vi "Data_Save_summary.vi"(8 "Data in":T1, 11 "AllControls In":T2) -> (2 "数组":string[](array[string]), 3 "dup path":path)   [LabVIEW 2017]
uses:
  Ctrls/AllControls.ctl
  Ctrls/CSV_Data.ctl
  Ctrls/PathChoose.ctl
  <vilib>/Utility/file.llb/Write Delimited Spreadsheet (string).vi
  <vilib>/Utility/file.llb/Read Delimited Spreadsheet (string).vi
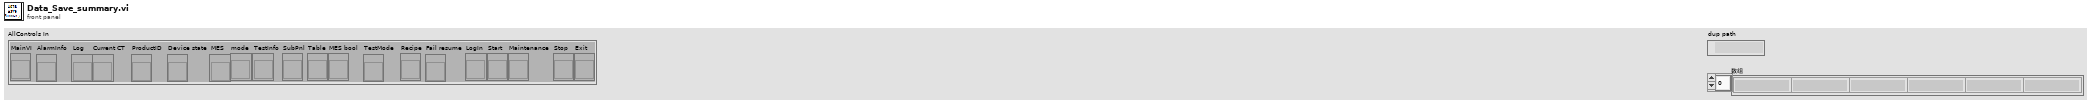
[diagram p1: front panel]
types:
  T1 = typedef "CSV_Data.ctl" = cluster{"SN":string, "Table":string[][], "Count":cluster{"Total":i32, "OK":i32, "NG":i32, "Yield":dbl}, "Start Time":timestamp, "daemon reference":refnum<k5>, "CT":dbl, "OK/NG":bool, "Station ID":string, "MES DDM SN":string, "MES PCBA SN":string, "Retest":string, "Attachment RFID detection":cluster{"UID":string, "tag content":string}, "SKU":string, "Plate_Diameter":string, "Alarm":string}
  T2 = typedef "AllControls.ctl" = cluster{"MainVI":refnum<vi>, "AlarmInfo":refnum<vi>, "Log":refnum<vi>, "Current CT":refnum<vi>, "ProductID":refnum<vi>, "Device state":refnum<vi>, "MES":refnum<vi>, "mode":refnum<vi>, "TestInfo":refnum<vi>, "SubPnl":refnum<vi>, "Table":refnum<vi>, "MES bool":refnum<vi>, "TestMode":refnum<vi>, "Recipe":refnum<vi>, "Fail resume":refnum<vi>, "LogIn":refnum<vi>, "Start":refnum<vi>, "Maintenance":refnum<vi>, "Stop":refnum<vi>, "Exit":refnum<vi>}
  T3 = typedef "PathChoose.ctl" = enum16{"OperatorLog", "AutoRunLog", "AlmLog", "TestData", "AllTestData", "backup_nvm", "backup_before_flashing"}
  T4 = enum16{"open", "replace", "create", "open or create", "replace or create", "replace or create with confirmation"}
  T5 = typedef "TesterInfo.ctl" = cluster{"Station Name":string, "Station Code":string, "ES NO.":string, "Tester ID":string, "PassMark Revision":string, "Rig ID":string, "Deamon_vision":string, "Project Name":string, "FFTesterPath":path, "Enable_User":bool, "Mode":enum16{"682"}, "MES":bool}
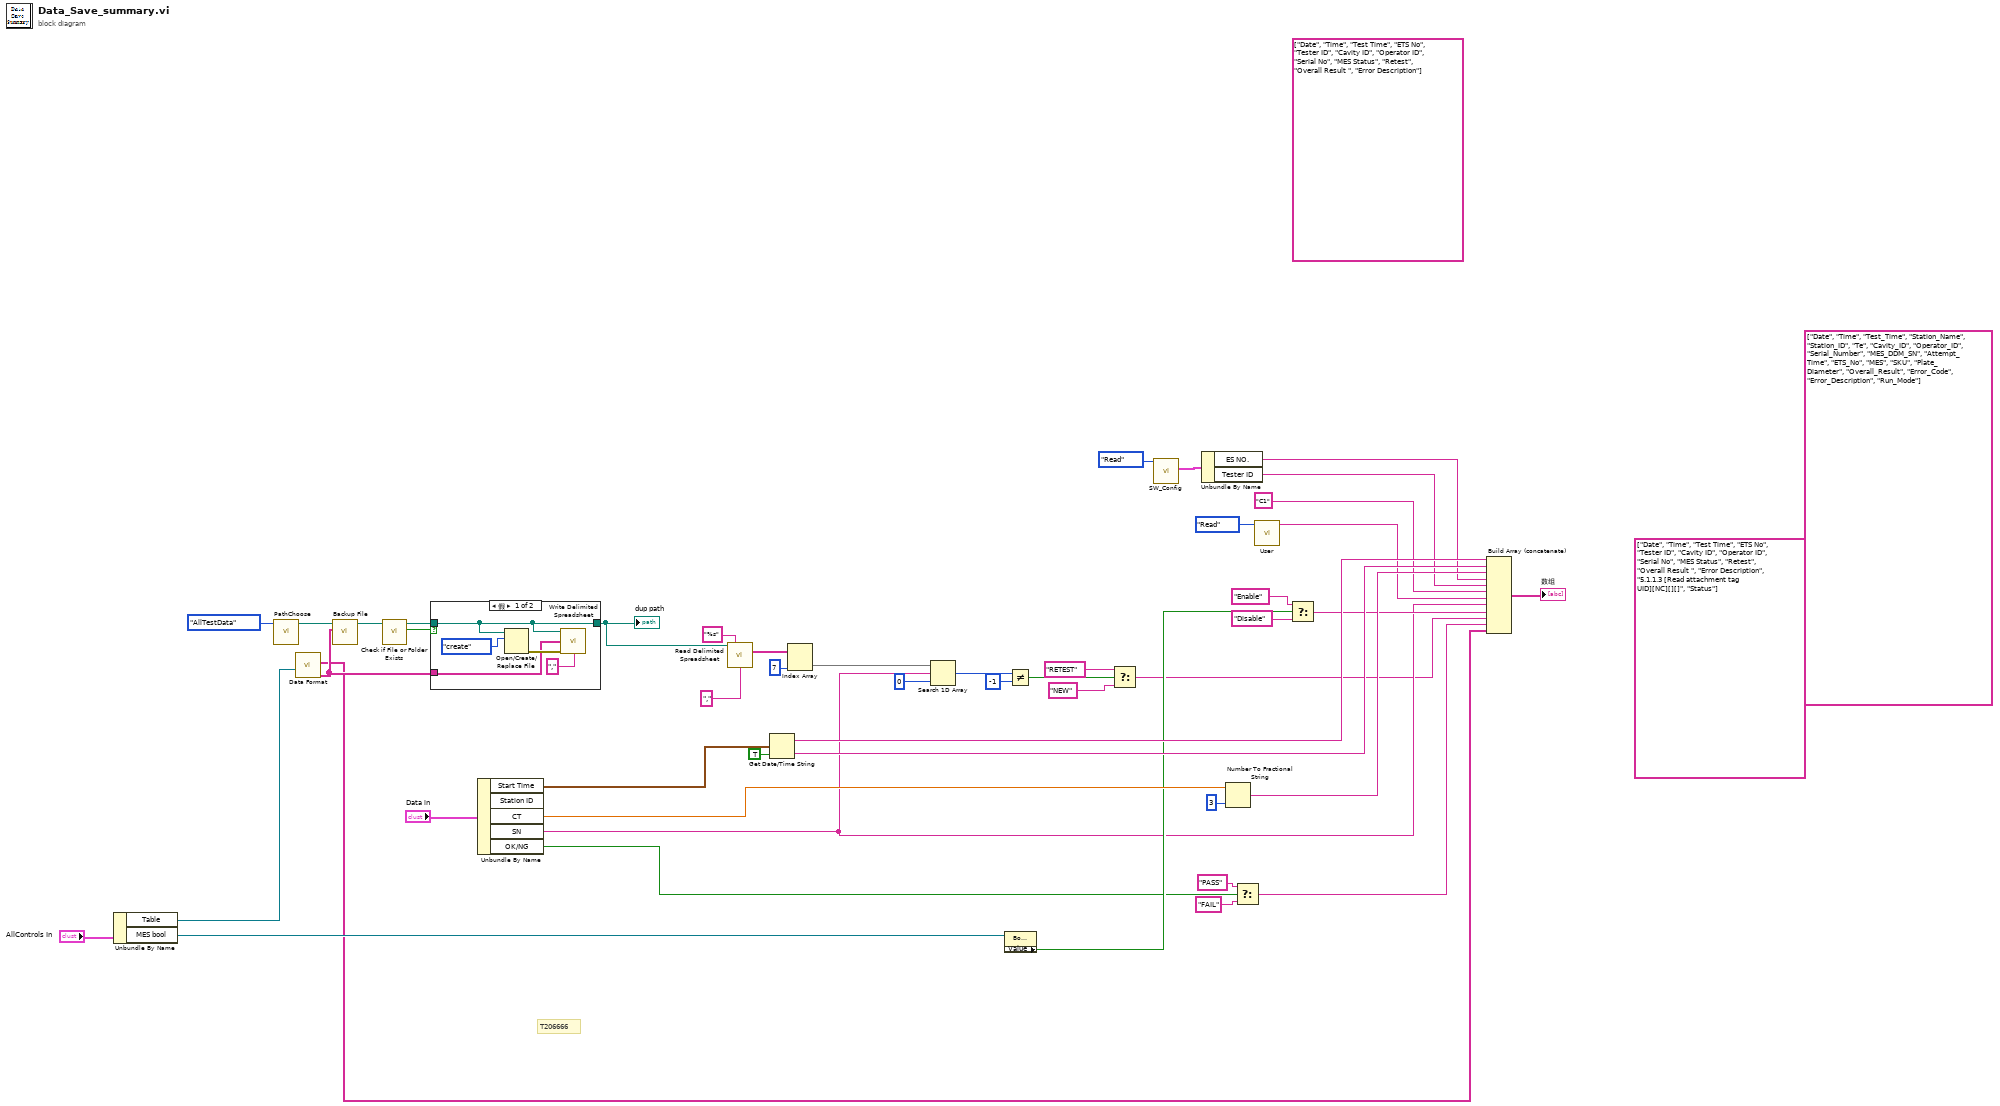
[diagram p0: block diagram]
diagram:
  (unwired) string[] ["Date", "Time", "Test Time", "ETS No", "Tester ID", "Cavity ID", "Operator ID", "Serial No", "MES Status", "Retest", "Overall Result ", "Error Description", "5.1.1.3 [Read attachment tag UID][NC][][]", "Status"] ("title")
  (unwired) string[] ["Date", "Time", "Test Time", "ETS No", "Tester ID", "Cavity ID", "Operator ID", "Serial No", "MES Status", "Retest", "Overall Result ", "Error Description"] ("title")
  (unwired) string[] ["Date", "Time", "Test_Time", "Station_Name", "Station_ID", "Te", "Cavity_ID", "Operator_ID", "Serial_Number", "MES_DDM_SN", "Attempt_Time", "ETS_No", "MES", "SKU", "Plate_Diameter", "Overall_Result", "Error_Code", "Error_Description", "Run_Mode"]
  # "T206666"
  n1 = Unbundle By Name("AllControls In") -> ("Table"=w2:refnum<vi>, "MES bool"=w41:refnum<vi>)
  n2 = call "PathChoose.vi"(11:PathChoose."AllTestData") -> ("Path_Out"=w39:path)  [unwired: 10 in]
  n3 = call "Data Format.vi"("Table"=w2) -> ("title"=w36:string[], "Data"=w1:string[])  [unwired: 9 in]
  n4 = call "Backup File.vi"("列首字符串"=w36, "path"=w39) -> ("path 2"=w38:path)  [unwired: 9 in]
  n5 = call <vilib>:"Check if File or Folder Exists.vi"("path"=w38) -> ("file or folder exists?"=w47:bool, "dup path"=w46:path)  [unwired: 8 in, 1 out]
  n6 = case shown="假" w47 {
    tunnel: w46 -> [w51 w54]
    tunnel: [w51 w54] -> w13
    tunnel: w36 -> [w49 _]
    frame False {
      n7 = Open/Create/Replace File(file path (use dialog)=w51, operation (0:open)=T4."create") -> (error out=w50:errorcluster)  [unwired: 4 in, 2 out]
      n8 = call-poly <vilib>:"Write Delimited Spreadsheet.vi"("file path (dialog if empty)"=w51, "1D data"=w49, "error in (no error)"=w50, "delimiter (\\t)"="," ("delimiter (\\t)")) -> ()  [unwired: 10 in, 2 out]
    }
    frame True {
    }
  }
  "dup path" <- w13
  n9 = Unbundle By Name("Data in") -> ("Start Time"=w35:timestamp, "CT"=w43:dbl, "SN"=w11:string, "OK/NG"=w18:bool)  [unwired: 1 out]
  n10 = call-poly <vilib>:"Read Delimited Spreadsheet.vi"("file path (dialog if empty)"=w13, "format (%s)"="%s" ("format (%.3f)"), "delimiter (\\t)"="," ("delimiter (\\t)")) -> ("all rows"=w15:string[][])  [unwired: 7 in, 5 out]
  n11 = Get Date/Time String(seconds (now)=w35, want seconds? (F)=TRUE ("需要秒？(F)")) -> (date string=w34:string, time string=w33:string)  [unwired: 1 in]
  n12 = Index Array(array=w15, index (col)=7 ("disabled index (col)")) -> (element=w12:string[])  [unwired: 1 in]
  n13 = Search 1D Array(1D array=w12, element=w11, start index (0)=0) -> (index of element=w10:i32)
  n14 = property class="Bool (严格)"(reference=w41) -> ("Value"=w21:bool)  [unwired: 1 in, 2 out]
  n15 = Not Equal?(x=w10, y=-1) -> (x != y?=w7:bool)
  n16 = Select(t="RETEST" ("element"), s=w7, f="NEW" ("element")) -> (s? t:f=w4:string)
  n17 = call "SW_Config.vi"("Step"=enum16{"Initial", "Write", "Read"}."Read") -> ("SW Config out"=w30:T5)  [unwired: 9 in, 1 out]
  n18 = Unbundle By Name(w30) -> ("ES NO."=w29:string, "Tester ID"=w28:string)
  n19 = Number To Fractional String(number=w43, precision (6)=i16 3 ("精度(6)")) -> (F-format string=w32:string)  [unwired: 2 in]
  n20 = Select(t="PASS" ("真字符串"), s=w18, f="FAIL" ("假字符串")) -> (s? t:f=w3:string)
  n21 = call "User.vi"("Step"=enum16{"Initial", "Write", "Read"}."Read") -> ("User out"=w26:string)  [unwired: 9 in, 1 out]
  n22 = Select(t="Enable" ("element"), s=w21, f="Disable") -> (s? t:f=w23:string)
  n23 = Build Array (concatenate)(w34, w33, w32, w29, w28, "C1" ("element"), w26, w11, w23, w4, w3, w1) -> (→"数组":string[])
